vi "Test Find All Variables.vi"() -> (0 "error out":errorcluster, 2 "Array":string[](array[string]))   [LabVIEW 2014, in "Scan Engine tests.lvlib"]
uses:
  Scan Engine tests.lvlib
  <vilib>/NI/Tag Bus/tag/tag descriptor.lvclass/tag descriptor.ctl
  editor node/Scan Engine editor node.lvclass
  <vilib>/NI/Tag Bus/tag/tag descriptor.lvclass
panel:
  out "path":path
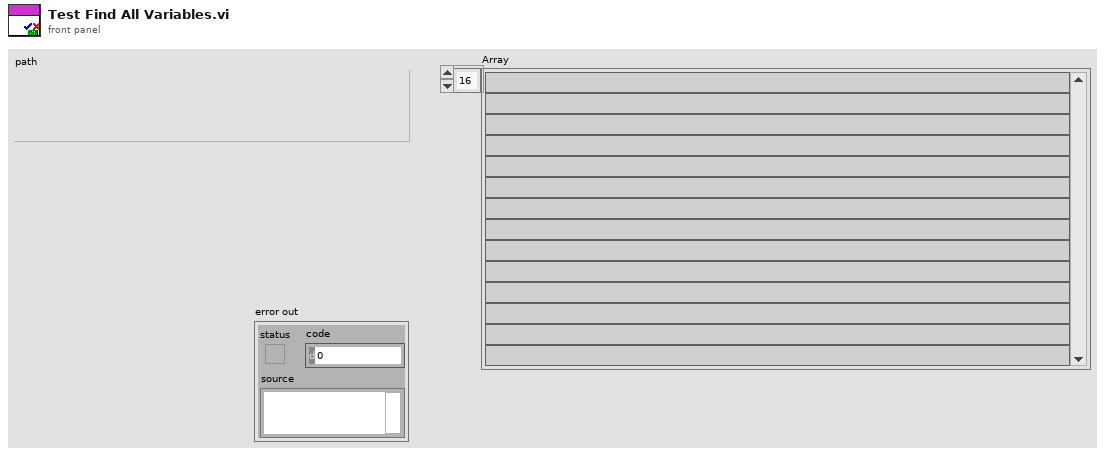
[diagram p1: front panel]
types:
  T1 = typedef "Scan Engine configuration.lvclass/Line.ctl" = cluster{"channel":refnum<class "TBM channel.lvclass">, "Tag":string}
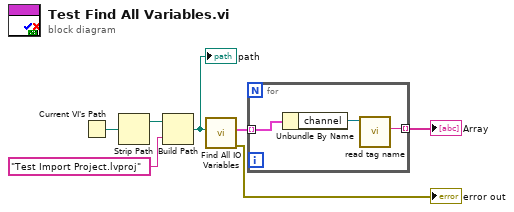
[diagram p0: block diagram]
diagram:
  n1 = Current VI's Path() -> (path=w5:path)
  n2 = Strip Path(path=w5) -> (stripped path=w4:path)  [unwired: 1 out]
  n3 = Build Path(base path=w4, name or relative path="Test Import Project.lvproj") -> (appended path=w2:path)
  "path" <- w2
  n4 = call "Find All IO Variables.vi"("Path"=w2) -> ("error out"=→"error out":errorcluster, "Tags"=w7:T1[])  [unwired: 9 in]
  n5 = for {
    tunnel: w7 -> [w10] mode=indexing
    tunnel: [w8] -> w6 mode=indexing
    n6 = Unbundle By Name(w10) -> ("channel"=w9:refnum<class "TBM channel.lvclass">)
    n7 = call <vilib>:"read tag name.vi"("system tag in"=w9) -> ("name"=w8:string)  [unwired: 8 in, 2 out]
  }
  "Array" <- w6
